vi "ReadUser.vi"() -> (1 "数组":string[](array[string]), 2 "文本":string, 3 "添加的路径":path)   [LabVIEW 2018]
uses:
  Global.vi
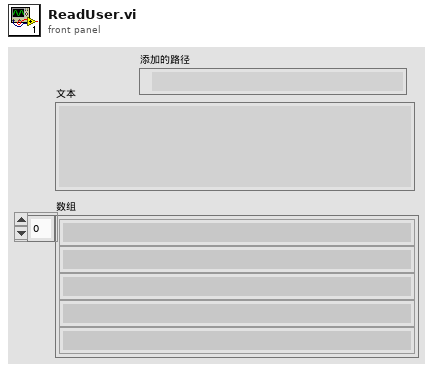
[diagram p1: front panel]
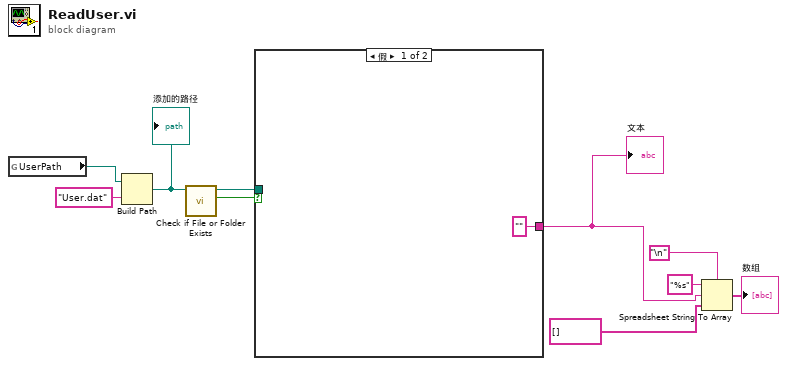
[diagram p0: block diagram]
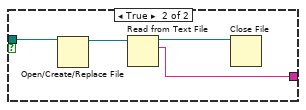
[diagram p2: hidden frame]
diagram:
  n1 = global read "Global.vi" "UserPath"() -> (w10:path)
  n2 = Build Path(base path=w10, name or relative path="User.dat" ("名称或相对路径")) -> (appended path=w8:path)
  "添加的路径" <- w8
  n3 = call <vilib>:"Check if File or Folder Exists.vi"("path"=w8) -> ("file or folder exists?"=w7:bool, "dup path"=w6:path)  [unwired: 8 in, 1 out]
  n4 = case shown="假" w7 {
    tunnel: w6 -> [_ w15]
    tunnel: ["" w12] -> w3
    frame False {
    }
    frame True {
      n5 = Open/Create/Replace File(file path (use dialog)=w15) -> (refnum out=w14:refnum<file>)  [unwired: 5 in, 2 out]
      n6 = Read from Text File(file (use dialog)=w14) -> (refnum out=w13:refnum<file>, text=w12:string)  [unwired: 3 in, 2 out]
      n7 = Close File(refnum=w13) -> ()  [unwired: 1 in, 2 out]
    }
  }
  "文本" <- w3
  n8 = Spreadsheet String To Array(delimiter (Tab)="\n", format string="%s" ("格式字符串"), spreadsheet string=w3, array type (2D Dbl)=string[] []) -> (array=→"数组":string[])
